vi "InitializePattern.vi"(8 "error in (no error)":errorcluster, 10 "Parameters":T1={"number of planes"=4, "z step"=1.9999999999999998e-05, "pixel dwell time"=1.0000000000000001e-11, "z frequency"=10.0, "number of pixels"=100, "smooth points"=10, "smooth line"=10, "Sine\nSawtooth"=FALSE, "PointSorting"=0, "Sort Points"=FALSE, "X-pixels"=256.0, "Y-lines"=256.0, "pixelstoµm"=256.0, "zoom"=1.0, "Time offset"=1.0000000000000001e-11} {"zoom" min=0.5 step=0.1; "Y-lines" min=1 step=1; "X-pixels" min=1 step=1; "PointSorting" items=["No Difference", "Every Second Point", "Down / Up"]; "smooth line" min=1; "smooth points" min=1; "number of pixels" min=1; "z frequency" format="%_4g"; "number of planes" min=1}, 11 "XYZ Point coordinates Pattern (pixels)":dbl[][](array[numeric])) -> (0 "error out":errorcluster, 1 "Parameters":T1={"number of planes"=4, "z step"=1.9999999999999998e-05, "pixel dwell time"=1.0000000000000001e-11, "z frequency"=10.0, "number of pixels"=100, "smooth points"=10, "smooth line"=10, "Sine\nSawtooth"=FALSE, "PointSorting"=0, "Sort Points"=FALSE, "X-pixels"=256.0, "Y-lines"=256.0, "pixelstoµm"=256.0, "zoom"=1.0, "Time offset"=1.0000000000000001e-11} {"zoom" min=0.5 step=0.1; "Y-lines" min=1 step=1; "X-pixels" min=1 step=1; "PointSorting" items=["No Difference", "Every Second Point", "Down / Up"]; "smooth line" min=1; "smooth points" min=1; "number of pixels" min=1; "z frequency" format="%_4g"; "number of planes" min=1}, 2 "DutyCluster":T2 {"Iteration" items=["first iteration", "second iteration"]}, 3 "Point coordinates (µm)":dbl[][](array[numeric]))   [LabVIEW 2010]
uses:
  TypeDefs/DutyCluster.ctl
  TypeDefs/ParameterCluster.ctl
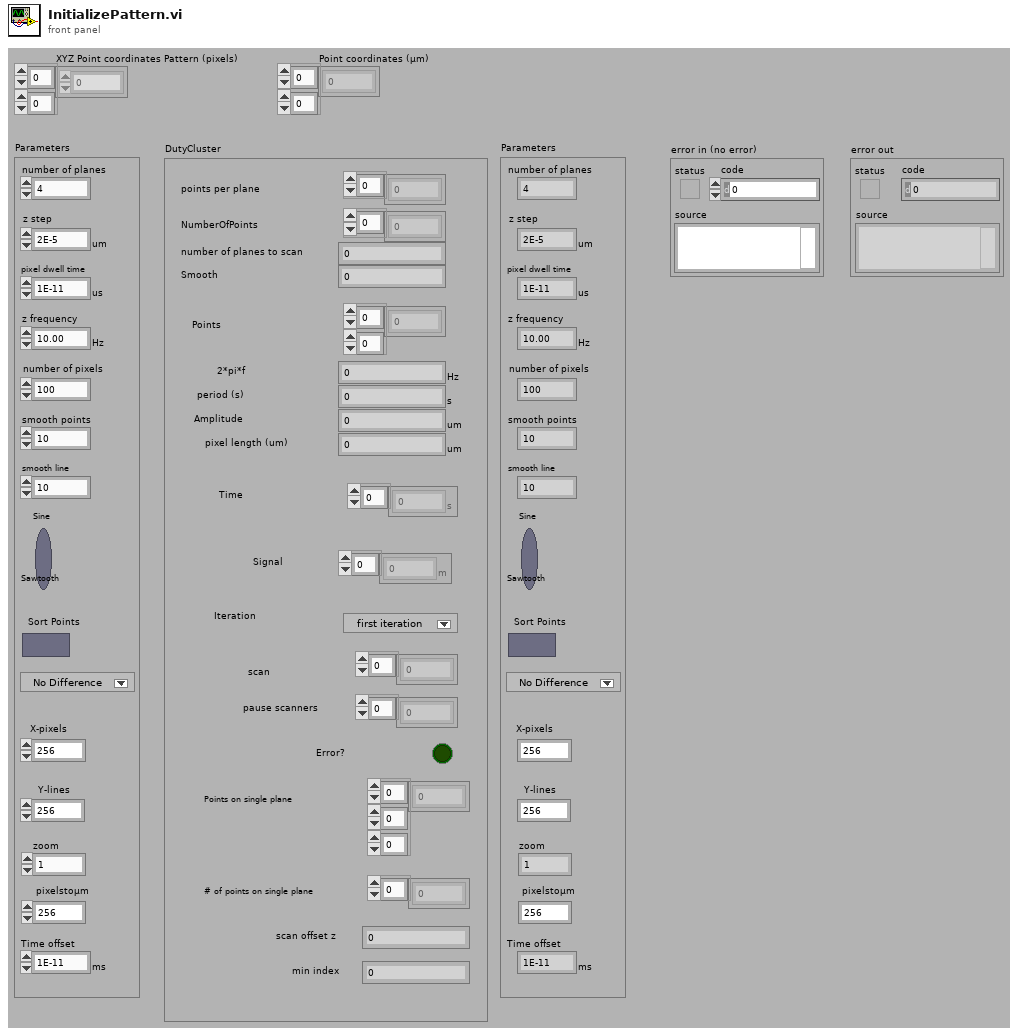
[diagram p1: front panel]
types:
  T1 = typedef "ParameterCluster.ctl" = cluster{"number of planes":i32, "z step":dbl[unit], "pixel dwell time":dbl[unit], "z frequency":dbl[unit], "number of pixels":i32, "smooth points":i32, "smooth line":i32, "Sine\nSawtooth":bool, "PointSorting":u16, "Sort Points":bool, "X-pixels":sgl, "Y-lines":sgl, "pixelstoµm":dbl, "zoom":dbl, "Time offset":dbl[unit]}
  T2 = typedef "DutyCluster.ctl" = cluster{"points per plane":i32[], "NumberOfPoints":i32[], "number of planes to scan":i32, "Smooth":i32, "Points":dbl[][], "2*pi*f":dbl[unit], "period (s)":dbl[unit], "Amplitude":dbl[unit], "pixel length (um)":dbl[unit], "Time":dbl[unit][], "Signal":dbl[unit][], "Iteration":u16, "scan":i32[], "pause scanners":i32[], "Error?":bool, "Points on single plane":dbl[][][], "# of points on single plane":i32[], "scan offset z":i32, "min index":i32}
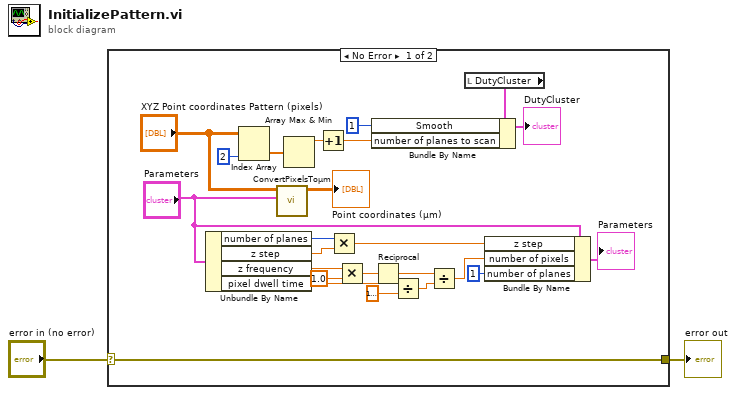
[diagram p0: block diagram]
diagram:
  n1 = case shown="No Error" "error in (no error)" {
    selector: "error in (no error)" -> [w17 w27]
    tunnel: [w17 w27] -> w1
    frame No Error {
      n2 = Unbundle By Name("Parameters") -> ("number of planes"=w15:i32, "z step"=w14:dbl[unit], "z frequency"=w5:dbl[unit], "pixel dwell time"=w7:dbl[unit])
      n3 = Index Array(array="XYZ Point coordinates Pattern (pixels)", index (col)=2 ("disabled index (col)")) -> (element=w25:dbl[])  [unwired: 1 in]
      n4 = call "ConvertPixelsToµm.vi"("Parameters"="Parameters", "Point coordinates (pixels)"="XYZ Point coordinates Pattern (pixels)") -> ("Point coordinates (µm)"=→"Point coordinates (µm)":dbl[][])  [unwired: 6 in, 1 out]
      n5 = Array Max & Min(array=w25) -> (max value=w24:dbl)  [unwired: 3 out]
      n6 = Increment(x=w24) -> (x+1=w19:dbl)
      n7 = Multiply(x=w15, y=w14) -> (x*y=w13:dbl[unit])
      n8 = Multiply(x=w5, y=dbl[unit] 1.0) -> (x*y=w4:dbl)
      n9 = Reciprocal(x=w4) -> (1/x=w12:dbl)
      n10 = Divide(x=w7, y=dbl[unit] 1e-06) -> (x/y=w6:dbl)
      n11 = Divide(x=w12, y=w6) -> (x/y=w11:dbl)
      n12 = local read "DutyCluster"() -> (w22:T2)
      n13 = Bundle By Name(cluster=w22, "Smooth"=1, "number of planes to scan"=w19) -> (→"DutyCluster":T2)
      n14 = Bundle By Name(cluster="Parameters", "z step"=w13, "number of pixels"=w11, "number of planes"=1) -> (→"Parameters":T1)
    }
    frame Error {
    }
  }
  "error out" <- w1
